vi "hasSoundStarted.vi"(8 "error in (no error)":errorcluster, 11 "BECHWCBasic in":refnum<class "BECHWCBasic.lvclass">) -> (0 "error out":errorcluster, 2 "started?":bool, 3 "BECHWCBasic out":refnum<class "BECHWCBasic.lvclass">)   [LabVIEW 2011, in "Hardware.lvlib" / "HWControllers.lvlib" / "BECHWCBasic.lvclass"]
uses:
  BECHWCBasic.lvclass
  BECHWCBasic.lvclass/BECHWCBasic.ctl
  Channels/Digital/DigitalOutput.lvclass
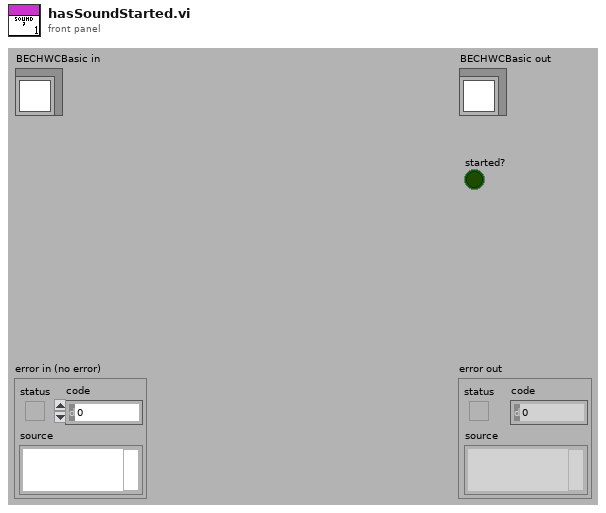
[diagram p1: front panel]
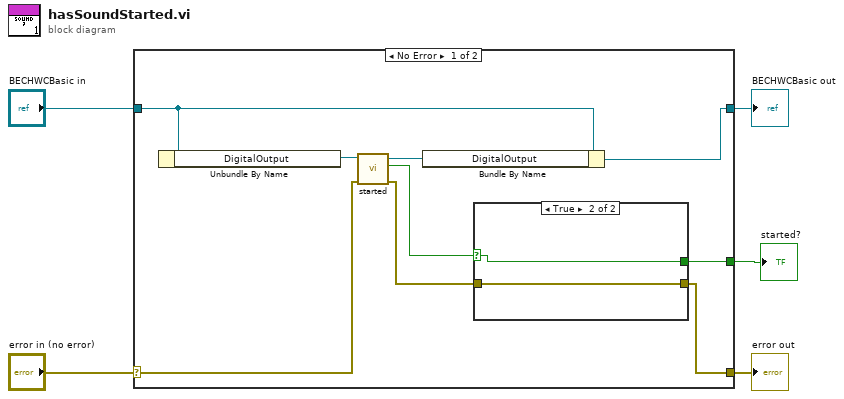
[diagram p0: block diagram]
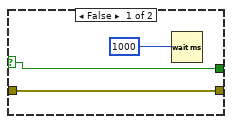
[diagram p2: hidden frame]
diagram:
  n1 = case shown="No Error" "error in (no error)" {
    selector: "error in (no error)" -> [w10 w21]
    tunnel: [w7 w21] -> w4
    tunnel: [w12 w20] -> w2
    tunnel: "BECHWCBasic in" -> [w13 w20]
    tunnel: [w6 _] -> w1
    frame No Error {
      n2 = Unbundle By Name(w13) -> ("DigitalOutput"=w14:refnum<class "DigitalOutput.lvclass">)
      n3 = call-dynamic "started.vi"("error in (no error)"=w10, "DigitalOutput in"=w14) -> ("error out"=w8:errorcluster, "started?"=w9:bool, "DigitalOutput out"=w11:refnum<class "DigitalOutput.lvclass">)  [unwired: 7 in]
      n4 = Bundle By Name(cluster=w13, "DigitalOutput"=w11) -> (w12:refnum<class "BECHWCBasic.lvclass">)
      n5 = case shown="True" w9 {
        selector: w9 -> [w15 w18]
        tunnel: w8 -> [w16 w19]
        tunnel: [w16 w19] -> w7
        tunnel: [w15 w18] -> w6
        frame False {
          n6 = Wait (ms)(milliseconds to wait=1000) -> ()  [unwired: 1 out]
        }
        frame True {
        }
      }
    }
    frame Error {
    }
  }
  "error out" <- w4
  "BECHWCBasic out" <- w2
  "started?" <- w1
